vi "Compact Acquisition Software.vi"() -> ()   [LabVIEW 2022 SP3]
uses:
  Controls/All Notifer.ctl
  Controls/UI Data.ctl
  Controls/Config.ctl
  Controls/Root path.ctl
  Controls/All Loop Status.ctl
  9a3150e6-56cf-486d-8976-296f0c56f58a.vi
  f5995a21-5467-4d79-ba42-6401d0487c2b.vi
  b49e865f-9608-438f-8b3f-50d1ceeb6397.vi
  2ab09cd3-f6ad-46c6-8934-8ba6e9181128.vi
  0b75de06-b87c-40eb-ad5f-27e6ba161dd7.vi
  df10829c-ba2f-467a-a207-c0f13a0d0a80.vi
  Sub VI's/Global 1.vi
  <vilib>/Utility/TDMS File Viewer/NI_TDMS File Viewer.lvlib
panel:
  out "trans2":bool
  in  "AO Tab":enum32{"Page 1", "Page 2"}(tab)
  in  "AO_1":dbl
  in  "AO_2":dbl min=-10.0 max=10.0
  in  "AO_3":dbl
  in  "AO_4":dbl
  in  "AO_5":dbl
  in  "AO_6":dbl
  in  "AO_7":dbl caption="AO_3"
  in  "AO_8":dbl caption="AO_4"
  in  "Exit":bool
  out "transparent":bool
  in  "Tab Control":T1(tab)
  in  "tdms":bool
  in  "SEQ":bool
  in  "File transfer":T2={"File status"=FALSE, "sent file"=FALSE, "Remote Path"="/home/lvuser/natinst/bin/startup.rtexe", "Password"="", "user@host"="admin@1.1.1.4", "Local File Path"=path ""}
  in  "Enter Time(period)":dbl=15.0 format="%#_g min"
  in  "Target IP Address:":string="169.254.219.4"
  in  "RT connect":bool
  out "Device Name":string
  in  "*Select Hardware Configuration File":string(combo)
  in  "Activate Task":T3
  out "ACC,TC,SG 2":waveform(dbl)[](graph) caption="PT & RTD"
  out "ACC,TC,SG":waveform(dbl)[](graph) caption="Thermocouple Graph"
  out "HSS 10":bool
  out "HSS 9":bool
  out "HSS 8":bool
  out "HSS 7":bool
  out "HSS 6":bool
  out "HSS 5":bool
  out "HSS 4":bool
  out "HSS 3":bool
  out "HSS 2":bool
  out "HSS 1":bool
  in  "Valve_10":bool caption="EPV_10"
  in  "Valve_ 9":bool caption="EPV_9"
  in  "Valve_ 8":bool caption="EPV_8"
  in  "Valve_ 7":bool caption="EPV_7"
  in  "Valve_ 6":bool caption="EPV_6"
  in  "Valve_ 5":bool caption="EPV_5"
  in  "Valve_ 4":bool caption="EPV_4"
  in  "Valve_ 3":bool caption="EPV_3"
  in  "Valve_ 2":bool caption="EPV_2"
  in  "Valve_1":bool
  out "AI_ 10":dbl caption="AI_10" format="%#.3g bar"
  out "AI_ 9":dbl caption="AI_9" format="%#.3g bar"
  out "AI_ 8":dbl caption="AI_8" format="%#.3g bar"
  out "AI_ 7":dbl caption="AI_7" format="%#.3g bar"
  out "AI_ 6":dbl caption="AI_6" format="%#.3g bar"
  out "AI_ 5":dbl caption="AI_5" format="%#.3g bar"
  out "AI_ 4":dbl caption="HE_RTD_ATF_7" format="%#.3g Kelvin"
  out "AI_ 3":dbl caption="He_PT_ATF_1" format="%#.3g Volt"
  out "AI_ 2":dbl caption="M_RTD_1" format="%#.3g kelvin"
  out "AI_1":dbl caption="AI_3" format="%#.3g V"
  out "TC_10":dbl caption="CHN_10" format="%#.3g Deg C"
  out "TC_9":dbl caption="CHN_9" format="%#.3g Deg C"
  out "TC_8":dbl caption="CHN_8" format="%#.3g Deg C"
  out "TC_7":dbl caption="CHN_7" format="%#.3g Deg C"
  out "TC_6":dbl caption="CHN_6" format="%#.3g Deg C"
  out "TC_5":dbl caption="CHN_5" format="%#.3g Deg C"
  out "TC_4":dbl caption="CHN_4" format="%#.3g Deg C"
  out "TC_3":dbl caption="CHN_3" format="%#.3g Deg C"
  out "TC_2":dbl caption="CHN_2" format="%#.3g Deg C"
  out "TC1":dbl caption="CHN_1" format="%#.3g Deg C"
  in  "Select type":u16(ring) items=["Thermocouple", "Accelerometer", "Strain Gauge"]
  out "RT health":bool caption="RT Health"
  in  "Datalog Title:":string
  in  "Start DAQ":bool
  in  "Start Datalog":bool
  out "Data Logging?":bool
  out "SG":bool
  out "ACC":bool
  out "DI":bool
  out "TC":bool
  out "DO":bool
  out "AO":bool
  out "AI":bool
  out "Time Stamp":timestamp format="%<%x %.X>T"
  in  "Update AO":bool
  in  "Listbox":i32(listbox)
  out "vi reference":refnum<vi>
  # "Compact Acquisition Software Version 1.0"
  # "Agnikul Cosmos Private Ltd,Chennai."
  # "Analog outputs \n(1-4) channels)"
  # "Analog outputs \n(5-8)channels)"
  # "1.Select the task on the \"Activate task palette\" to perform the selected Acquisition.\n2.Select Hardware configuration File.\nTo create a new configuration,click on the \"Hardware configuration\"\nbutton in the left corner list.\n3.Start DAQ.\n4.Enter Datalog Name.\n5.Start Datalog."
  # "Every datalog will Restart at the user \ndefined time period.\n\"Default Restart time is 15 minutes.\""
  # "*Note:User Can configure 10 Analog inputs,8 Analog Outputs,10 Digital inputs,10 Digital Outputs\n10 Strain Gauge,10 Accelerometer and 10 Thermocouple."
  # "HOME"
  # "HARDWARE COFIGURATION"
  # "Digital Outputs & inputs\n (Max 10 channels)"
  # "Analog inputs\n(Max 10 channels)"
  # "TEST MODE"
  # "Help"
  # "Help and Support"
  # "If you have any doubts please contact us(Software development team)."
  # "Contact us"
  # "-Get in touch with us"
  # "Contact Info\nSoftware Development Team-LabVIEW\nEmail:\nVigneshwaranc@agnikul.in\nKannansolai@agnikul.in\nParikshitmandvikar@agnikul.in\nAjaikumar@agnikul.in"
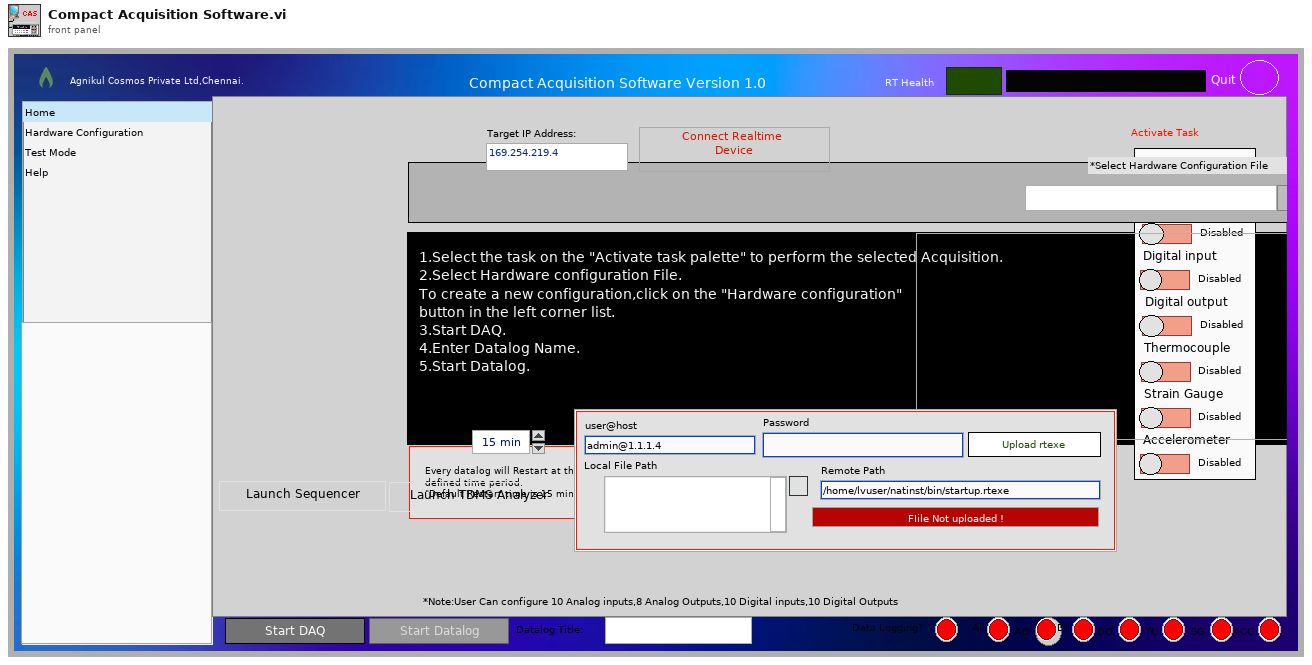
[diagram p1: front panel]
types:
  T1 = enum32{"Home Page", "Hardware Configuration", "Test Mode", "Graph View"}
  T2 = cluster{"File status":bool, "sent file":bool, "Remote Path":string, "Password":string, "user@host":string, "Local File Path":path}
  T3 = cluster{"Analog input":bool, "Analog Output":bool, "Digital input":bool, "Digital output":bool, "Thermocouple":bool, "Strain Gauge":bool, "Accelerometer":bool}
  T4 = enum32{"invalid app kind", "Development System", "Run Time System", "Student Edition", "Embedded LabVIEW", "Evaluation", "Custom"}
  T5 = typedef "All Notifer.ctl" = cluster{"UI Data":refnum<notifier>, "Start DAQ":refnum<notifier>, "Start Log":refnum<notifier>}
  T6 = typedef "Config.ctl" = cluster{"AO config":cluster{"Channel_Name":string, "Channel_Number":string, "Default_Value":dbl, "Units":string}[], "AI config":cluster{"Channel_Name":string, "Channel_Number":string, "Pre_Scale_min":dbl, "Pre_Scale_max":dbl, "Sensor_min":dbl, "Sensor_max":dbl, "Units":string}[], "DI config":cluster{"Channel_Name":string, "Channel_Number":string, "Default_Value":bool, "DI invert?":bool}[], "DO config":cluster{"Channel_Name":string, "Channel_Number":string, "Default_Value":bool, "DO invert?":bool}[], "TC config":cluster{"Channel_Name":string, "Channel_Number":string, "Pre_Scale_min":dbl, "Pre_Scale_max":dbl, "units":i32, " type":i32}[], "ACC config":cluster{"Channel_Name":string, "Channel_Number":string, "Pre_Scale_min":dbl, "Pre_Scale_max":dbl, "Terminal configuration":i32, "Sensitivity":dbl, "Sensitivity units":i32}[], "SG config":cluster{"Channel_Name":string, "Channel_Number":string, "Pre_Scale_min":dbl, "Pre_Scale_max":dbl}[], "Strain Gauge Settings":cluster{"poisson ratio":dbl, "nominal gage resistance":dbl, "gage factor":dbl}, "bridge information":cluster{"strain configuration":i32, "lead wire resistance":dbl, "initial bridge voltage":dbl, "voltage excitation source":i32, "voltage excitation value":dbl}, "Sample Rate":cluster{"AI Sample Rate":dbl, "AO Sample Rate":dbl, "DI Sample Rate":dbl, "TC Sample Rate":dbl, "DO Sample Rate":dbl, "SG Sample Rate":dbl, "ACC Sample Rate":dbl}}
  T7 = typedef "Root path.ctl" = cluster{"Data":path, "Sub VI's":path, "Source code":path}
  T8 = cluster{"notifiers ref":T5, "DAQ ref":cluster{"DI ref":refnum<vi>[], "DO ref":refnum<vi>[], "AI ref":refnum<vi>[], "AO ref":refnum<vi>[], "SG,TC,ACC":refnum<vi>[]}, "Config":T6, "NO.of.DO":u8, "NO.of.AO":u8, "user event out":refnum<user-event>, "Channel names":cluster{"AO Names":string[], "AI Names":string[], "DI Names":string[], "DO Names":string[], "TC Names":string[], "AO Default":dbl[], "DO Default":bool[], "ACC Names":string[], "SG Names":string[]}, "AO,AI,DI,DO,TC,ACC,SG":i32[], "CDAQ/CRIO(T)":bool, "DO value":bool[], "AO Value":dbl[], "Ctrl ref":cluster{"Start DAQ":refnum<vi>, "Start Log":refnum<vi>, "Tab Control":refnum<vi>}, "Root Path":T7}
  T9 = enum16{"Init", "EnQ '1'", "EnQ 'n'", "EnQ Opp", "DeQ", "Flush", "Close"}
  T10 = enum8{"Enabled", "Disabled", "Disabled and Grayed Out"}
  T11 = cluster{"no.of di":u8, "no.of ai":u8, "no.of do":u8, "no.of ao":u8, "no.of SG":u8}
  T12 = enum16{"Controls", "Transparents", "indicators", "Strings"}
  T13 = enum32{"Invalid", "Standard", "Closed", "Hidden", "Minimized", "Maximized"}
  T14 = cluster{"AO Names":string[], "AI Names":string[], "DI Names":string[], "DO Names":string[], "TC Names":string[], "AO Default":dbl[], "DO Default":bool[], "ACC Names":string[], "SG Names":string[]}
  T15 = cluster{"DI ref":refnum<vi>[], "DO ref":refnum<vi>[], "AI ref":refnum<vi>[], "AO ref":refnum<vi>[], "SG,TC,ACC":refnum<vi>[]}
  T16 = typedef "All Queue.ctl" = cluster{"AI\nAO\nDO\nTC\nACC\nStrain":refnum<queue>[], "DI":refnum<queue>}
  T17 = enum16{"Init", "Read 'All'", "Read 'n'", "Read '1'", "Write '1'", "Write 'n'", "Write 'All'"}
  T18 = cluster{"Activate Task":cluster{"Analog input":bool, "Analog Output":bool, "Digital input":bool, "Digital output":bool, "Thermocouple":bool, "Strain Gauge":bool, "Accelerometer":bool}, "Start DAQ":bool, "Start Time":timestamp, "DO Names":string[], "AO Names":string[], "AO Default":dbl[], "DO Default":bool[], "Config":cluster{"AO config":cluster{"Channel_Name":string, "Channel_Number":string, "Default_Value":dbl, "Units":string}[], "AI config":cluster{"Channel_Name":string, "Channel_Number":string, "Pre_Scale_min":dbl, "Pre_Scale_max":dbl, "Sensor_min":dbl, "Sensor_max":dbl, "Units":string}[], "DI config":cluster{"Channel_Name":string, "Channel_Number":string, "Default_Value":bool, "DI invert?":bool}[], "DO config":cluster{"Channel_Name":string, "Channel_Number":string, "Default_Value":bool, "DO invert?":bool}[], "TC config":cluster{"Channel_Name":string, "Channel_Number":string, "Pre_Scale_min":dbl, "Pre_Scale_max":dbl, "units":i32, " type":i32}[], "ACC config":cluster{"Channel_Name":string, "Channel_Number":string, "Pre_Scale_min":dbl, "Pre_Scale_max":dbl, "Terminal configuration":i32, "Sensitivity":dbl, "Sensitivity units":i32}[], "SG config":cluster{"Channel_Name":string, "Channel_Number":string, "Pre_Scale_min":dbl, "Pre_Scale_max":dbl}[], "Strain Gauge Settings":cluster{"poisson ratio":dbl, "nominal gage resistance":dbl, "gage factor":dbl}, "Bridge Settings":cluster{"voltage excitation value":dbl, "voltage excitation source":i32, "initial bridge voltage":dbl, "lead wire resistance":dbl, "strain configuration":i32}, "Sample Rate":cluster{"AI Sample Rate":dbl, "AO Sample Rate":dbl, "DI Sample Rate":dbl, "TC Sample Rate":dbl, "DO Sample Rate":dbl, "SG Sample Rate":dbl, "ACC Sample Rate":dbl}}}
  T19 = typedef "All Loop Status.ctl" = enum16{"AI", "AO", "DI", "DO", "TC", "Strain", "ACC", "RT", "Log", "Seq", "Sync"}
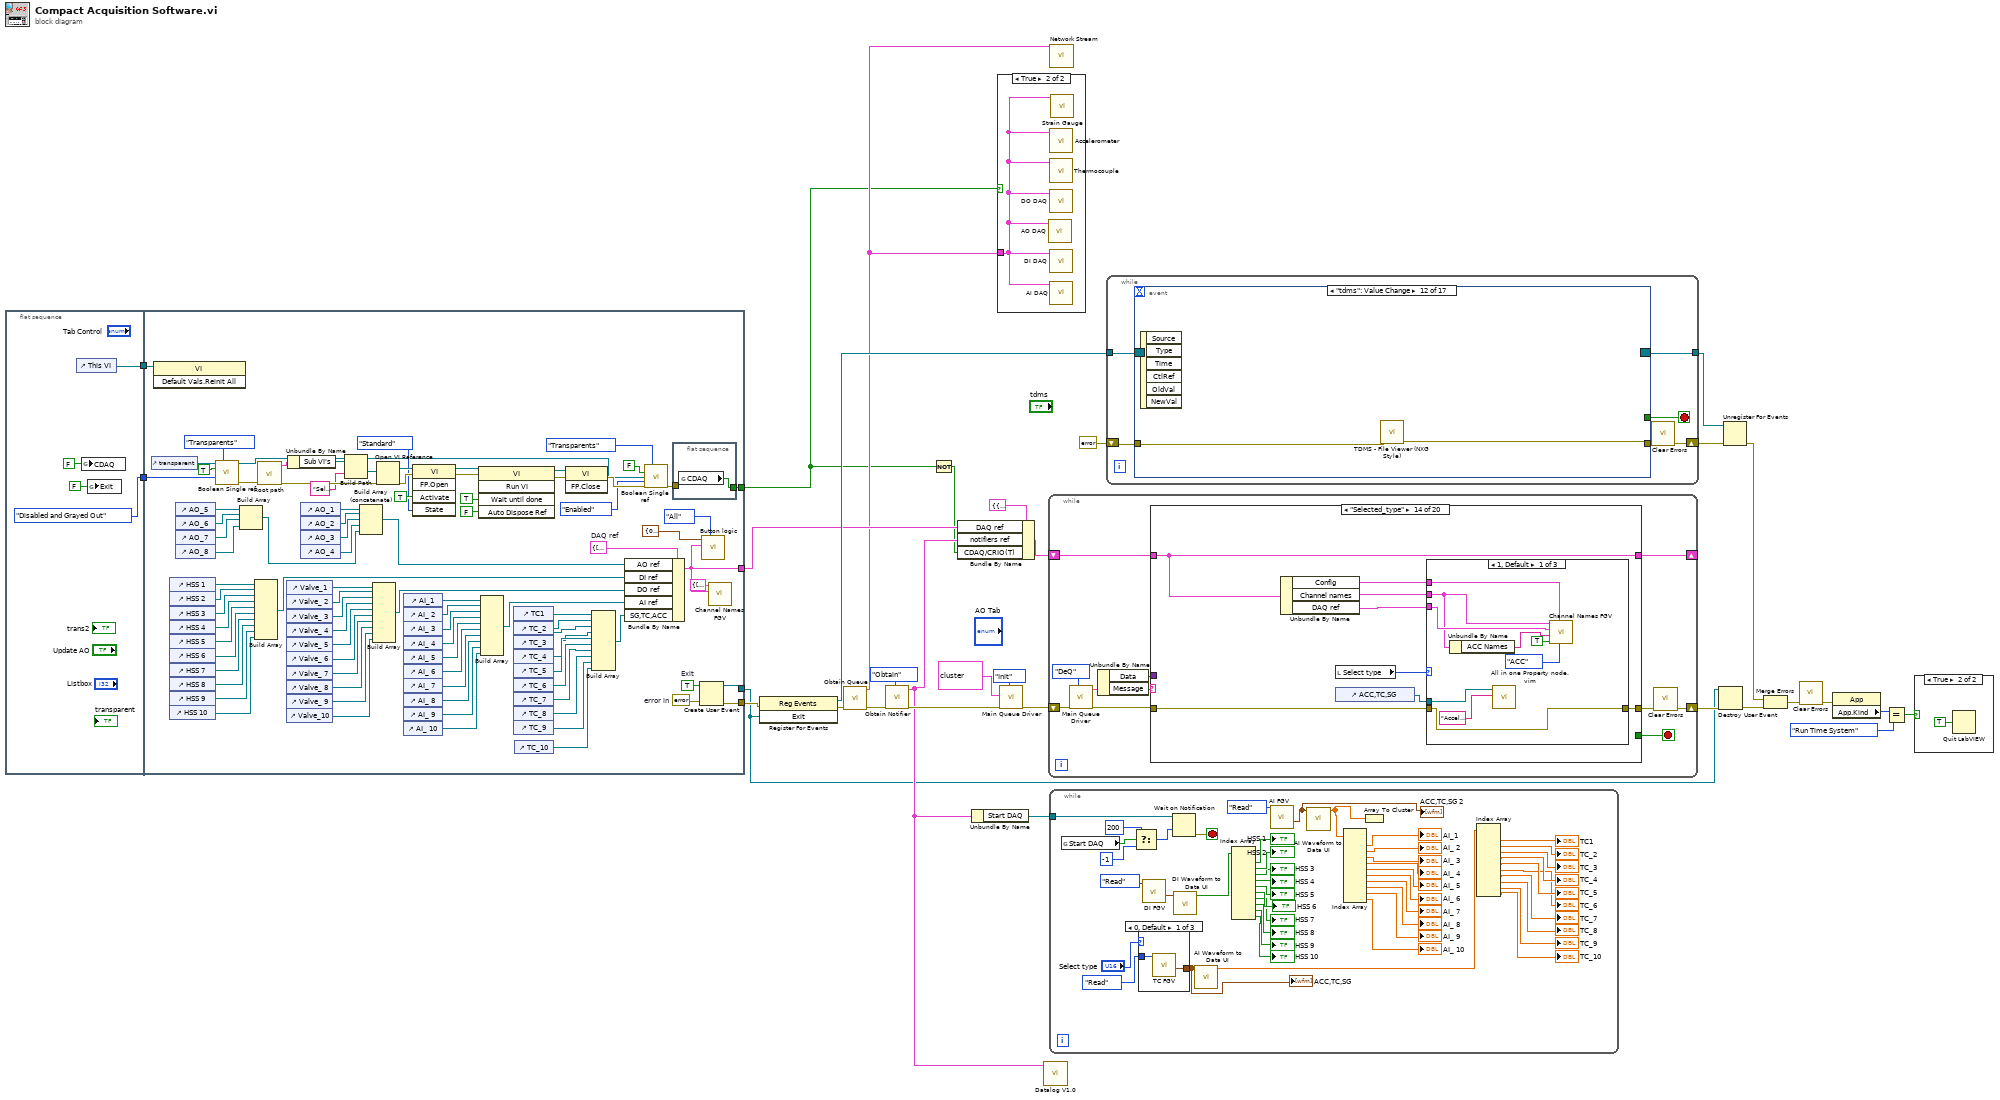
[diagram p0: block diagram]
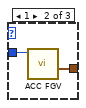
[diagram p4: hidden frame]
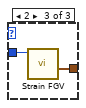
[diagram p5: hidden frame]
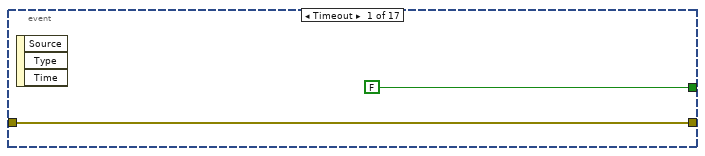
[diagram p6: hidden frame]
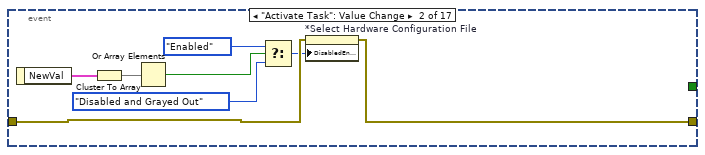
[diagram p7: hidden frame]
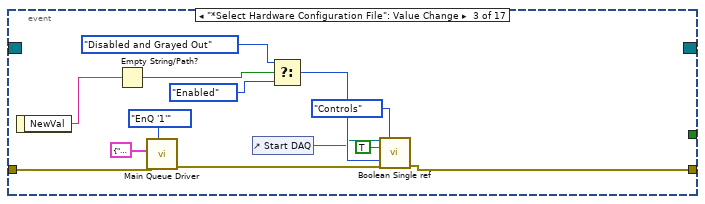
[diagram p8: hidden frame]
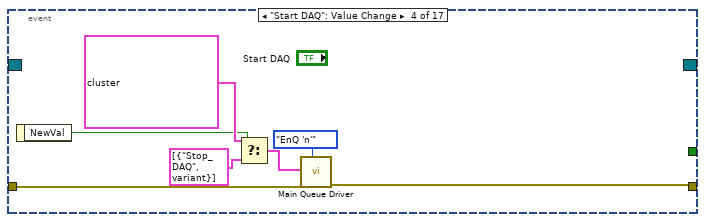
[diagram p9: hidden frame]
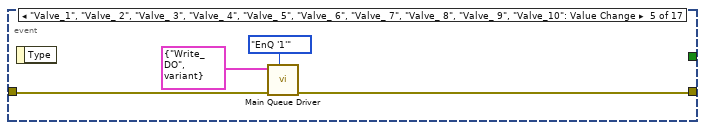
[diagram p10: hidden frame]
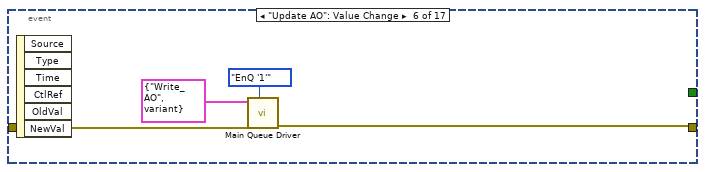
[diagram p11: hidden frame]
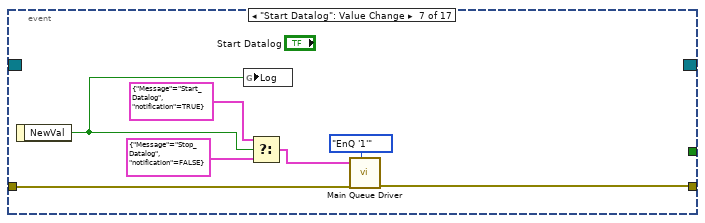
[diagram p12: hidden frame]
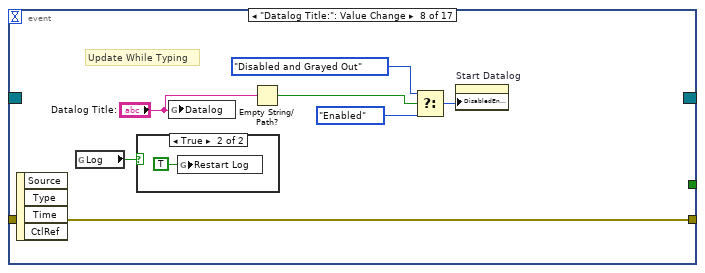
[diagram p13: hidden frame]
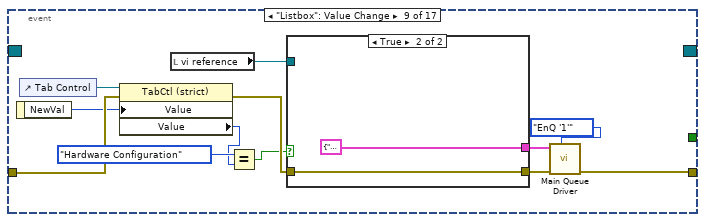
[diagram p15: hidden frame]
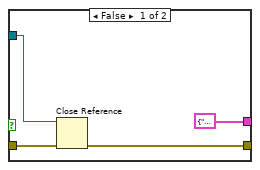
[diagram p16: hidden frame]
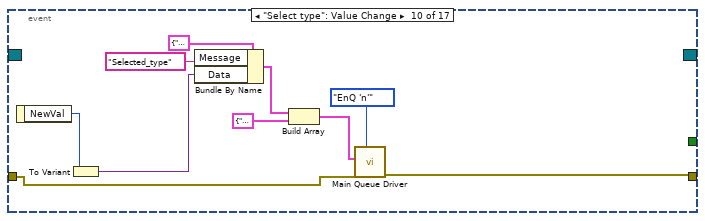
[diagram p17: hidden frame]
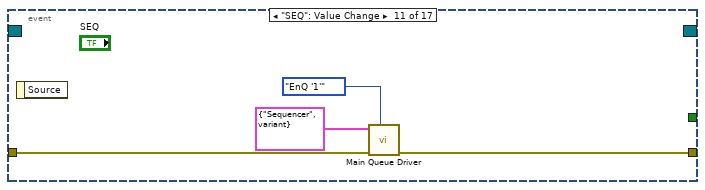
[diagram p18: hidden frame]
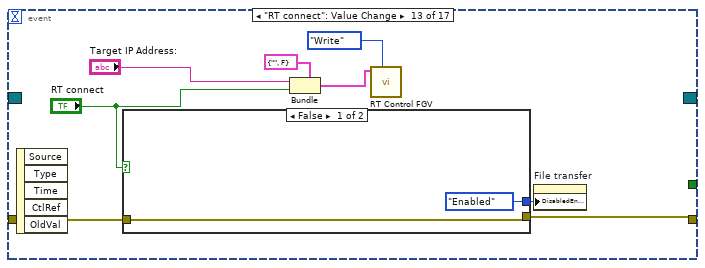
[diagram p19: hidden frame]
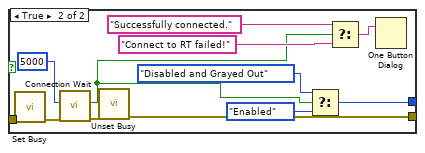
[diagram p20: hidden frame]
diagram:
  n1 = flat-sequence {
    tunnel: [w33] -> w12
    tunnel: [T10."Disabled and Grayed Out" ("Disabled")] -> w10
    tunnel: [w76] -> w18
    tunnel: [w57] -> w13
    tunnel: w12 -> [w54]
    tunnel: [w46] -> w1
    tunnel: [w45] -> w11
    tunnel: w10 -> [w43]
    frame #0 {
      n2 = control-ref of="This VI"() -> (w33:refnum<vi>)
      n3 = global write "Global 1.vi" "CDAQ"(FALSE ("CDAQ")) -> ()
      n4 = global write "Global 1.vi" "Exit"(FALSE ("Exit")) -> ()
    }
    frame #1 {
      w47 = TRUE  # Exit
      w44 = errorcluster {"status"=FALSE, "code"=0, "source"=""}  # error in
      w96 = T15 {"DI ref"=[], "DO ref"=[], "AI ref"=[], "AO ref"=[], "SG,TC,ACC"=[]}  # DAQ ref
      n5 = control-ref of="transparent"() -> (w64:refnum<vi>)
      n6 = invoke on="Invoke Node" class="VI" method="Default Vals.Reinit All"(reference=w54) -> ()  [unwired: 2 in, 3 out]
      n7 = control-ref of="HSS 1"() -> (w116:refnum<vi>)
      n8 = control-ref of="HSS 2"() -> (w115:refnum<vi>)
      n9 = control-ref of="HSS 3"() -> (w107:refnum<vi>)
      n10 = control-ref of="HSS 4"() -> (w114:refnum<vi>)
      n11 = control-ref of="HSS 5"() -> (w113:refnum<vi>)
      n12 = control-ref of="HSS 6"() -> (w112:refnum<vi>)
      n13 = control-ref of="HSS 7"() -> (w111:refnum<vi>)
      n14 = control-ref of="HSS 8"() -> (w110:refnum<vi>)
      n15 = control-ref of="HSS 9"() -> (w109:refnum<vi>)
      n16 = control-ref of="HSS 10"() -> (w108:refnum<vi>)
      n17 = control-ref of="AO_5"() -> (w40:refnum<vi>)
      n18 = control-ref of="AO_6"() -> (w39:refnum<vi>)
      n19 = control-ref of="AO_7"() -> (w38:refnum<vi>)
      n20 = control-ref of="AO_8"() -> (w37:refnum<vi>)
      n21 = call "Boolean Single ref.vi"("Enum"=T12."Transparents", "Visible"=TRUE, "trans"=w64, "Disabled"=w43) -> ("trans out"=w61:refnum<vi>, "error out"=w53:errorcluster)  [unwired: 9 in, 1 out]
      n22 = Build Array(w40, w39, w38, w37) -> (w36:refnum<vi>[])
      n23 = Build Array(w116, w115, w107, w114, w113, w112, w111, w110, w109, w108) -> (w95:refnum<vi>[])
      n24 = call "Root path.vi"("error in (no error)"=w53) -> ("error out"=w52:errorcluster, "Root Path"=w51:T7)  [unwired: 9 in]
      n25 = control-ref of="Valve_1"() -> (w126:refnum<vi>)
      n26 = control-ref of="Valve_ 2"() -> (w125:refnum<vi>)
      n27 = control-ref of="Valve_ 3"() -> (w124:refnum<vi>)
      n28 = control-ref of="Valve_ 4"() -> (w123:refnum<vi>)
      n29 = control-ref of="Valve_ 5"() -> (w122:refnum<vi>)
      n30 = control-ref of="Valve_ 6"() -> (w121:refnum<vi>)
      n31 = control-ref of="Valve_ 7"() -> (w120:refnum<vi>)
      n32 = control-ref of="Valve_ 8"() -> (w119:refnum<vi>)
      n33 = control-ref of="Valve_ 9"() -> (w118:refnum<vi>)
      n34 = control-ref of="Valve_10"() -> (w117:refnum<vi>)
      n35 = Unbundle By Name(w51) -> ("Sub VI's"=w50:path)
      n36 = control-ref of="AO_1"() -> (w92:refnum<vi>)
      n37 = control-ref of="AO_2"() -> (w91:refnum<vi>)
      n38 = control-ref of="AO_3"() -> (w90:refnum<vi>)
      n39 = control-ref of="AO_4"() -> (w89:refnum<vi>)
      n40 = Build Path(base path=w50, name or relative path="Select Device.vi") -> (appended path=w48:path)
      n41 = Build Array (concatenate)(w92, w91, w90, w89, w36) -> (w88:refnum<vi>[])
      n42 = Build Array(w126, w125, w124, w123, w122, w121, w120, w119, w118, w117) -> (w94:refnum<vi>[])
      n43 = Open VI Reference(vi path=w48, error in (no error)=w52) -> (vi reference=w69:refnum<vi>, error out=w70:errorcluster)  [unwired: 4 in]
      n44 = control-ref of="AI_1"() -> (w106:refnum<vi>)
      n45 = control-ref of="AI_ 2"() -> (w105:refnum<vi>)
      n46 = control-ref of="AI_ 3"() -> (w104:refnum<vi>)
      n47 = control-ref of="AI_ 4"() -> (w103:refnum<vi>)
      n48 = control-ref of="AI_ 5"() -> (w102:refnum<vi>)
      n49 = control-ref of="AI_ 6"() -> (w101:refnum<vi>)
      n50 = control-ref of="AI_ 7"() -> (w100:refnum<vi>)
      n51 = control-ref of="AI_ 8"() -> (w99:refnum<vi>)
      n52 = control-ref of="AI_ 9"() -> (w98:refnum<vi>)
      n53 = control-ref of="AI_ 10"() -> (w97:refnum<vi>)
      n54 = invoke on="Invoke Node" class="VI" method="FP.Open"(reference=w69, error in=w70, "Activate"=TRUE ("Activate?"), "State"=T13."Standard") -> (reference out=w71:refnum<vi>, error out=w72:errorcluster)  [unwired: 1 in, 3 out]
      n55 = invoke on="Invoke Node" class="VI" method="Run VI"(reference=w71, error in=w72, "Wait until done"=TRUE ("Wait Until Done"), "Auto Dispose Ref"=FALSE ("Auto Dispose Reference")) -> (reference out=w73:refnum<vi>, error out=w74:errorcluster)  [unwired: 1 in, 3 out]
      n56 = Build Array(w106, w105, w104, w103, w102, w101, w100, w99, w98, w97) -> (w93:refnum<vi>[])
      n57 = control-ref of="TC1"() -> (w87:refnum<vi>)
      n58 = control-ref of="TC_2"() -> (w78:refnum<vi>)
      n59 = control-ref of="TC_3"() -> (w79:refnum<vi>)
      n60 = control-ref of="TC_4"() -> (w80:refnum<vi>)
      n61 = control-ref of="TC_5"() -> (w81:refnum<vi>)
      n62 = control-ref of="TC_6"() -> (w86:refnum<vi>)
      n63 = control-ref of="TC_7"() -> (w85:refnum<vi>)
      n64 = control-ref of="TC_8"() -> (w84:refnum<vi>)
      n65 = control-ref of="TC_9"() -> (w83:refnum<vi>)
      n66 = control-ref of="TC_10"() -> (w82:refnum<vi>)
      n67 = invoke on="Invoke Node" class="VI" method="FP.Close"(reference=w73, error in=w74) -> (error out=w62:errorcluster)  [unwired: 1 in, 2 out]
      n68 = Build Array(w87, w78, w79, w80, w81, w86, w85, w84, w83, w82) -> (w77:refnum<vi>[])
      n69 = Bundle By Name(cluster=w96, "AO ref"=w88, "DI ref"=w95, "DO ref"=w94, "AI ref"=w93, "SG,TC,ACC"=w77) -> (w76:T15)
      n70 = call "Boolean Single ref.vi"("Enum"=T12."Transparents", "Visible"=FALSE, "trans"=w61, "Disabled"=T10."Enabled", "error in (no error)"=w62) -> ("error out"=w58:errorcluster)  [unwired: 8 in, 2 out]
      n71 = flat-sequence {
        tunnel: w58 -> [_]
        tunnel: [w127] -> w57
        frame #0 {
          n72 = global read "Global 1.vi" "CDAQ"() -> (w127:bool)
        }
      }
      n73 = Create User Event(user event datatype=w47, error in=w44) -> (user event=w46:refnum<user-event>, error out=w45:errorcluster)
      n74 = call "Button logic.vi"("Enum"=enum16{"DI", "AI", "DO", "All", "SG"}."All", "DAQ ref"=w76, "Cluster"=T11 {"no.of di"=0, "no.of ai"=0, "no.of do"=0, "no.of ao"=0, "no.of SG"=0}) -> ()  [unwired: 9 in]
      n75 = call "Channel Names FGV.vi"("DAQ ref"=w76, "Channel names 2"=T14 {"AO Names"=["AO_1", "AO_2", "AO_3", "AO_4"], "AI Names"=["AI_1", "AI_2", "AI_3", "AI_4", "AI_5", "AI_6", "AI_7", "AI_8", "AI_9", "AI_10"], "DI Names"=[], "DO Names"=["EPV_1", "EPV_2", "EPV_3", "EPV_4", "EPV_5", "EPV_6", "EPV_7", "EPV_8", "EPV_9", "EPV_10"], "TC Names"=["CHN_1", "CHN_2", "CHN_3", "CHN_4", "CHN_5", "CHN_6", "CHN_7", "CHN_8", "CHN_9", "CHN_10"], "AO Default"=[], "DO Default"=[], "ACC Names"=[], "SG Names"=[]}) -> ()  [unwired: 10 in]
    }
  }
  n76 = register-events(error in=w11, w1) -> (reference out=w29:refnum<event-registration>, error out=w21:errorcluster)  [unwired: 1 in]
  n77 = call "Obtain Queue.vi"("error in"=w21) -> ("error out"=w20:errorcluster, "Queue ref"=w15:T16)  [unwired: 9 in]
  n78 = call "Obtain Notifier.vi"("Case"=enum16{"Obtain", "Read"}."Obtain", "error in (no error)"=w20) -> ("error out"=w23:errorcluster, "notifiers out"=w16:T5)  [unwired: 8 in]
  n79 = Not(x=w13) -> (.not. x?=w14:bool)
  n80 = Bundle By Name(cluster=T8 {"notifiers ref"={"UI Data"=refnum, "Start DAQ"=refnum, "Start Log"=refnum}, "DAQ ref"={"DI ref"=[], "DO ref"=[], "AI ref"=[], "AO ref"=[], "SG,TC,ACC"=[]}, "Config"={"AO config"=[], "AI config"=[], "DI config"=[], "DO config"=[], "TC config"=[{"Channel_Name"="", "Channel_Number"="", "Pre_Scale_min"=0.0, "Pre_Scale_max"=0.0, "units"=4, " type"=7}], "ACC config"=[], "SG config"=[], "Strain Gauge Settings"={"poisson ratio"=0.3, "nominal gage resistance"=120.0, "gage factor"=2.08}, "bridge information"={"strain configuration"=10271, "lead wire resistance"=1.7, "initial bridge voltage"=0.0, "voltage excitation source"=10200, "voltage excitation value"=3.3}, "Sample Rate"={"AI Sample Rate"=0.0, "AO Sample Rate"=0.0, "DI Sample Rate"=0.0, "TC Sample Rate"=0.0, "DO Sample Rate"=0.0, "SG Sample Rate"=0.0, "ACC Sample Rate"=0.0}}, "NO.of.DO"=0, "NO.of.AO"=0, "user event out"=refnum, "Channel names"={"AO Names"=[], "AI Names"=[], "DI Names"=[], "DO Names"=[], "TC Names"=[], "AO Default"=[], "DO Default"=[], "ACC Names"=[], "SG Names"=[]}, "AO,AI,DI,DO,TC,ACC,SG"=[], "CDAQ/CRIO(T)"=TRUE, "DO value"=[], "AO Value"=[], "Ctrl ref"={"Start DAQ"=refnum, "Start Log"=refnum, "Tab Control"=refnum}, "Root Path"={"Data"=path "", "Sub VI's"=path "", "Source code"=path ""}}, "DAQ ref"=w18, "notifiers ref"=w16, "CDAQ/CRIO(T)"=w14) -> (w24:T8)
  n81 = Unbundle By Name(w16) -> ("Start DAQ"=w22:refnum<notifier>)
  n82 = case shown="True" w13 {
    tunnel: w15 -> [_ w128]
    frame False {
    }
    frame True {
      n83 = call "AO DAQ.vi"("Queue ref"=w128) -> ()  [unwired: 11 in]
      n84 = call "Accelerometer.vi"("Queue ref"=w128) -> ()  [unwired: 11 in]
      n85 = call "Thermocouple.vi"("Queue ref"=w128) -> ()  [unwired: 11 in]
      n86 = call "DO DAQ.vi"("Queue ref"=w128) -> ()  [unwired: 11 in]
      n87 = call "DI DAQ.vi"("Queue ref"=w128) -> ()  [unwired: 11 in]
      n88 = call "AI DAQ.vi"("Queue ref"=w128) -> ()  [unwired: 11 in]
      n89 = call "Strain Gauge.vi"("Queue ref"=w128) -> ()  [unwired: 11 in]
    }
  }
  n90 = call "Main Queue Driver.vi"("Option"=T9."Init", "error in (no error)"=w23, "Messages"=cluster{"Message":string, "Data":variant}[] [{"Message"="Initialize", "Data"=variant}, {"Message"="Login", "Data"=variant}, {"Message"="Refresh_files", "Data"=variant}]) -> ("error out"=w31:errorcluster)  [unwired: 7 in, 1 out]
  n91 = call "Datalog V1.0.vi"("notifiers in"=w16) -> ()  [unwired: 11 in]
  n92 = while {
    shift-right: [w139] -> w27
    shift-left: w31 -> [w131]
    shift-right: [w132] -> _
    shift-left: w24 -> [w133]
    stop <- w137 stop-if-true
    n93 = call "Main Queue Driver.vi"("Option"=T9."DeQ", "error in (no error)"=w131) -> ("error out"=w130:errorcluster, "Message Out"=w135:cluster{"Message":string, "Data":variant})  [unwired: 8 in]
    n94 = Unbundle By Name(w135) -> ("Data"=w129:variant, "Message"=w134:string)
    n95 = case shown="\"Selected_type\"" w134 {
      tunnel: w130 -> [w144 w166 w186 w207 w213 w233 w257 w271 w311 w324 w337 w369 w394 w402 w435 w441 w453 w458 w459 w478]
      tunnel: [w143 w163 w186 w207 w212 w225 w246 w268 w312 w325 w338 w367 w394 w401 w432 w440 w456 w458 w460 w480] -> w138
      tunnel: [_ FALSE _ _ _ _ _ _ _ _ _ _ _ _ _ _ _ _ _ TRUE] -> w137
      tunnel: w133 -> [w142 w176 w200 w206 w211 w218 w250 w265 w318 w330 w341 w370 w391 w399 w436 w438 w455 w457 w470 w484]
      tunnel: [w142 w180 w199 w206 w211 w227 w253 w266 w318 w330 w339 w371 w389 w399 w436 w438 w455 w457 w470 w484] -> w132
      tunnel: w129 -> [_ _ _ _ _ _ _ _ _ _ _ _ _ _ _ _ w451 _ _ _]
      frame "pollevent", Default {
        w156 = T19[] [enum."AI", enum."AO", enum."DI", enum."DO", enum."TC", enum."ACC", enum."Strain", enum."Log", enum."RT"] items=["AI", "AO", "DI", "DO", "TC", "Strain", "ACC", "RT", "Log", "Seq", "Sync"] ("Loops")
        n96 = Unbundle By Name(w142) -> ("DAQ ref.DO ref"=w141:refnum<vi>[], "DAQ ref.AO ref"=w140:refnum<vi>[])
        n97 = call "ALS Feedback DO ref.vi"("DAQ ref.AO ref"=w140, "DAQ ref.DO ref"=w141) -> ()  [unwired: 10 in]
        n98 = call "ALL Loop Status.vi"("Option"=T17."Read 'n'", "error in (no error)"=w144, "Loops"=w156) -> ("error out"=w143:errorcluster, "Status List Out"=w155:bool[])  [unwired: 6 in, 1 out]
        n99 = Index Array(array=w155) -> (element #1=→"AI":bool, element #2=→"AO":bool, element #3=→"DI":bool, element #4=→"DO":bool, element #5=→"TC":bool, element #6=→"ACC":bool, element #7=→"SG":bool, element #8=→"Data Logging?":bool, element #9=→"RT health":bool)  [unwired: 9 in]
        n100 = Get Date/Time In Seconds() -> (seconds since 1Jan1904=→"Time Stamp":timestamp)
      }
      frame "Initialize" {
        n101 = Unbundle By Name(w176) -> ("CDAQ/CRIO(T)"=w159:bool)
        n102 = property on="Listbox" class="LstBox (strict)"(error in=w166, "Item Names"=string[] ["Home", "Hardware Configuration", "Test Mode", "Help"]) -> (error out=w165:errorcluster)  [unwired: 1 in, 1 out]
        n103 = Select(t="Ready to Start Acquisition in Realtime (cRIO)" ("Device Name"), s=w159, f="Ready to Start Acquisition in cDAQ" ("Device Name")) -> (s? t:f=→"Device Name":string)
        n104 = control-ref of="RT health"() -> (w174:refnum<vi>)
        n105 = control-ref of="RT connect"() -> (w173:refnum<vi>)
        n106 = control-ref of="Target IP Address:"() -> (w160:refnum<vi>)
        n107 = global write "Global 1.vi" "ALS"(FALSE ("CDAQ")) -> ()
        n108 = Build Array(w174, w173, w160) -> (w172:refnum<vi>[])
        n109 = call "ALL Loop Status.vi"("Option"=T17."Init", "error in (no error)"=w165) -> ("error out"=w178:errorcluster)  [unwired: 7 in, 2 out]
        n110 = call "All in one Property node.vim"("Visible(T)/Value(F)"=TRUE ("Value(F)"), "Boolean"=w159, "ref in"=w172) -> ()  [unwired: 7 in, 2 out]
        n111 = property on="File transfer" class="Clust"("Visible"=w159) -> ()  [unwired: 2 in, 2 out]
        n112 = call "Root path.vi"("error in (no error)"=w178) -> ("error out"=w177:errorcluster, "Root Path"=w175:T7)  [unwired: 9 in]
        n113 = control-ref of="*Select Hardware Configuration File"() -> (w168:refnum<vi>)
        n114 = control-ref of="Tab Control"() -> (w179:refnum<vi>)
        n115 = control-ref of="Start DAQ"() -> (w171:refnum<vi>)
        n116 = control-ref of="Start Datalog"() -> (w170:refnum<vi>)
        n117 = property on="trans2" class="Bool (strict)"("Visible"=TRUE) -> ()  [unwired: 2 in, 2 out]
        n118 = Bundle By Name(cluster=w176, "Root Path"=w175, "Ctrl ref.Start DAQ"=w171, "Ctrl ref.Start Log"=w170, "Ctrl ref.Tab Control"=w179) -> (w180:T8)
        n119 = Build Array(w171, w170, w168) -> (w169:refnum<vi>[])
        n120 = call "All in one Property node.vim"("error in (no error)"=w177, "Boolean"=T10."Disabled and Grayed Out", "ref in"=w169) -> ("error out"=w163:errorcluster)  [unwired: 7 in, 1 out]
      }
      frame "Button Logic" {
        n121 = local read "Select type"() -> (w190:u16)
        n122 = Unbundle By Name(w200) -> ("DAQ ref"=w201:T15, "AO,AI,DI,DO,TC,ACC,SG"=w188:i32[])
        n123 = case shown="0" w190 {
          tunnel: [4 ("index") 5 ("index") 6 ("index")] -> w189
          frame 0 {
          }
          frame 1 {
          }
          frame 2, Default {
          }
        }
        n124 = To Unsigned Byte Integer(number=w188) -> (unsigned 8bit integer=w187:u8[])
        n125 = Index Array(array=w187, index #1=1 ("index"), index #5=w189) -> (element #1=w195:u8, element #2=w198:u8, element #3=w197:u8, element #4=w196:u8, element #5=w191:u8)  [unwired: 3 in]
        n126 = Bundle By Name(cluster=T11 {"no.of di"=0, "no.of ai"=0, "no.of do"=0, "no.of ao"=0, "no.of SG"=0} ("Cluster"), "no.of ao"=w195, "no.of ai"=w198, "no.of di"=w197, "no.of do"=w196, "no.of SG"=w191) -> (w202:T11)
        n127 = call "Button logic.vi"("Enum"=enum16{"DI", "AI", "DO", "All", "SG"}."All", "DAQ ref"=w201, "Cluster"=w202) -> ()  [unwired: 9 in]
        n128 = Bundle By Name(cluster=w200, "NO.of.DO"=w196, "NO.of.AO"=w195) -> (w199:T8)
      }
      frame "Login" {
      }
      frame "Refresh_files" {
        n129 = Unbundle By Name(w211) -> ("Root Path.Data"=w210:path)
        n130 = Build Path(base path=w210, name or relative path=path "HW config") -> (appended path=w208:path)
        n131 = List Folder(path=w208, error in=w213) -> (filenames=w215:string[], error out=w214:errorcluster)  [unwired: 2 in, 2 out]
        n132 = property on="*Select Hardware Configuration File" class="CmbBox"(error in=w214, "Strings[]"=w215) -> (error out=w212:errorcluster)  [unwired: 1 in, 1 out]
      }
      frame "Hardware_config" {
        n133 = Unbundle By Name(w218) -> ("Root Path.Sub VI's"=w217:path)
        n134 = Build Path(base path=w217, name or relative path=path "Hardware Config.vi") -> (appended path=w216:path)
        n135 = Open VI Reference(vi path=w216, error in (no error)=w233) -> (vi reference=w229:refnum<vi>, error out=w231:errorcluster)  [unwired: 4 in]
        "vi reference" <- w229
        n136 = flat-sequence {
          tunnel: [w239] -> w226
          tunnel: [w237] -> w220
          tunnel: w221 -> [w234]
          frame #0 {
            n137 = global read "Global 1.vi" "Hw file"() -> (w236:string)
            n138 = Empty String/Path?(string/path=w236) -> (empty?=w235:bool)
            n139 = case shown="False" w235 {
              tunnel: w236 -> [w243 _]
              tunnel: [w242 w244] -> w238
              tunnel: w234 -> [w241 w244]
              frame False {
                n140 = property on="*Select Hardware Configuration File" class="CmbBox"(error in=w241, "Val(Sgnl)"=w243) -> (error out=w242:errorcluster)  [unwired: 1 in, 1 out]
              }
              frame True {
              }
            }
            n141 = call "Config FGV.vi"("Enum"=enum16{"Read", "Write"}."Read", "error in (no error)"=w238) -> ("error out"=w237:errorcluster, "Data"=w239:T6)  [unwired: 8 in]
          }
        }
        n142 = invoke on="Sub Panel" class="SubPnl" method="Insert VI"(error in=w231, "VI Ref"=w229) -> (error out=w228:errorcluster)  [unwired: 2 in, 3 out]
        n143 = invoke on="Invoke Node" class="VI" method="Run VI"(reference=w229, error in=w228, "Wait until done"=FALSE ("Wait Until Done"), "Auto Dispose Ref"=FALSE ("Auto Dispose Reference")) -> (error out=w221:errorcluster)  [unwired: 1 in, 4 out]
        n144 = call "Main Queue Driver.vi"("Option"=T9."EnQ '1'", "Message"=cluster{"Message":string, "Data":variant} {"Message"="Refresh_files", "Data"=variant}) -> ("error out"=w224:errorcluster)  [unwired: 8 in, 1 out]
        n145 = Bundle By Name(cluster=w218, "Config"=w226) -> (w227:T8)
        n146 = Merge Errors(w220, w224, w221) -> (w225:errorcluster)
      }
      frame "Load_Config" {
        n147 = Unbundle By Name(w250) -> ("Root Path.Data"=w249:path)
        n148 = Build Path(base path=w249, name or relative path=path "HW config" ("Select Hardware Configuration File to Start DAQ")) -> (appended path=w247:path)
        n149 = Build Path(base path=w247, name or relative path="*Select Hardware Configuration File") -> (appended path=w251:path)
        n150 = call "Load Config.vi"("error in"=w257, "file path (use dialog)"=w251) -> ("error out"=w255:errorcluster, "data"=w254:T6)  [unwired: 8 in]
        n151 = call "Config FGV.vi"("Enum"=enum16{"Read", "Write"}."Write", "error in (no error)"=w255, "Data 2"=w254) -> ("error out"=w246:errorcluster, "Data"=w245:T6)  [unwired: 7 in]
        n152 = Bundle By Name(cluster=w250, "Config"=w245) -> (w253:T8)
      }
      frame "Start_DAQ" {
        n153 = Unbundle By Name(w265) -> ("CDAQ/CRIO(T)"=w264:bool, "Config"=w263:T6, "AO Value"=w262:dbl[], "DO value"=w261:bool[], "Ctrl ref.Tab Control"=w259:refnum<vi>)
        n154 = global write "Global 1.vi" "Start DAQ"(TRUE ("Start DAQ")) -> ()
        n155 = local write "Listbox"(2 ("Listbox")) -> ()
        n156 = property on="trans2" class="Bool (strict)"("Visible"=FALSE) -> ()  [unwired: 2 in, 2 out]
        n157 = call "All Channel Names.vi"("Enum"=enum16{"Read", "Write"}."Read") -> ("Channel names"=w270:T14)  [unwired: 13 in, 1 out]
        n158 = case shown="True" w264 {
          tunnel: "Activate Task" -> [w287 w305]
          tunnel: w265 -> [w275 w295]
          tunnel: w271 -> [w283 w307]
          tunnel: w270 -> [w282 w306]
          tunnel: [w278 w294] -> w268
          tunnel: [w275 w295] -> w266
          tunnel: w263 -> [_ w298]
          tunnel: w262 -> [_ w297]
          tunnel: w261 -> [_ w296]
          tunnel: w259 -> [w273 w290]
          frame False {
            w285 = enum16{"Read", "Write", "Start time", "init"}."Start time" ("Enum")
            n159 = Unbundle By Name(w282) -> ("DO Names"=w280:string[], "AO Names"=w281:string[])
            n160 = call "Activated TAsk.vi"("Enum"=enum16{"Read", "Write"}."Write", "error in (no error)"=w283, "Activate Task"=w287) -> ("error out"=w279:errorcluster, "Start Time"=w284:timestamp)  [unwired: 6 in, 1 out]
            n161 = Unbundle By Name(w275) -> ("notifiers ref.Start DAQ"=w277:refnum<notifier>)
            n162 = call "AO FGV.vi"("Enum"=w285, "Start Time"=w284, "AO Channel Names"=w281) -> ()  [unwired: 7 in, 2 out]
            n163 = property on="Property Node" class="TabCtl (strict)"(reference=w273, "Value"=T1."Test Mode") -> ()  [unwired: 1 in, 2 out]
            n164 = call "DO FGV.vi"("Enum"=w285, "Start Time"=w284, "DO Channel Names"=w280) -> ()  [unwired: 6 in, 3 out]
            n165 = Send Notification(notification=TRUE, notifier=w277, error in (no error)=w279) -> (error out=w278:errorcluster)  [unwired: 1 out]
          }
          frame True {
            # "RT DAQ"
            n166 = Unbundle By Name(w306) -> ("DO Names"=w304:string[], "AO Names"=w303:string[])
            n167 = Get Date/Time In Seconds() -> (seconds since 1Jan1904=w302:timestamp)
            n168 = Add(x=w302, y=5.0) -> (x+y=w300:timestamp)
            n169 = Bundle By Name(cluster=T18 {"Activate Task"={"Analog input"=TRUE, "Analog Output"=TRUE, "Digital input"=TRUE, "Digital output"=TRUE, "Thermocouple"=FALSE, "Strain Gauge"=TRUE, "Accelerometer"=TRUE}, "Start DAQ"=TRUE, "Start Time"=timestamp(0 s since 1904-01-01), "DO Names"=[], "AO Names"=[], "AO Default"=[], "DO Default"=[], "Config"={"AO config"=[], "AI config"=[], "DI config"=[], "DO config"=[], "TC config"=[{"Channel_Name"="", "Channel_Number"="", "Pre_Scale_min"=0.0, "Pre_Scale_max"=0.0, "units"=4, " type"=7}], "ACC config"=[], "SG config"=[], "Strain Gauge Settings"={"poisson ratio"=0.3, "nominal gage resistance"=120.0, "gage factor"=2.08}, "Bridge Settings"={"voltage excitation value"=3.3, "voltage excitation source"=10200, "initial bridge voltage"=0.0, "lead wire resistance"=1.7, "strain configuration"=10271}, "Sample Rate"={"AI Sample Rate"=0.0, "AO Sample Rate"=0.0, "DI Sample Rate"=0.0, "TC Sample Rate"=0.0, "DO Sample Rate"=0.0, "SG Sample Rate"=0.0, "ACC Sample Rate"=0.0}}}, "DO Names"=w304, "AO Names"=w303, "Activate Task"=w305, "Start Time"=w300, "Start DAQ"=TRUE, "Config"=w298, "AO Default"=w297, "DO Default"=w296) -> (w310:T18)
            n170 = property on="Property Node" class="TabCtl (strict)"(reference=w290, "Value"=T1."Test Mode") -> ()  [unwired: 1 in, 2 out]
            n171 = Unbundle By Name(w295) -> ("notifiers ref.Start DAQ"=w291:refnum<notifier>)
            n172 = To Variant(anything=w310) -> (Variant=w309:variant)
            n173 = call "Networkstream UI Command.vi"("error in"=w307, "Data"=w309, "Message"="Start DAQ") -> ("error out"=w293:errorcluster)  [unwired: 8 in]
            n174 = Send Notification(notification=TRUE ("ignore previous (F)"), notifier=w291, error in (no error)=w293) -> (error out=w294:errorcluster)  [unwired: 1 out]
          }
        }
      }
      frame "Update_DO" {
        n175 = Unbundle By Name(w318) -> ("DAQ ref.DO ref"=w317:refnum<vi>[])
        n176 = call "All Channel Names.vi"("Enum"=enum16{"Read", "Write"}."Read") -> ("Channel names"=w315:T14)  [unwired: 13 in, 1 out]
        n177 = Unbundle By Name(w315) -> ("DO Default"=w314:bool[])
        n178 = for {
          tunnel: w317 -> [w321] mode=indexing
          tunnel: [w322] -> w313 mode=indexing
          tunnel: w314 -> [w320] mode=indexing
          tunnel: w311 -> [w319]
          n179 = call "All in one Property node.vim"("error in (no error)"=w319, "Boolean"=w320, "ref in"=w321) -> ("error out"=w322:errorcluster)  [unwired: 7 in, 1 out]
        }
        n180 = Merge Errors(w313, w311) -> (w312:errorcluster)
      }
      frame "Update_AO" {
        n181 = Unbundle By Name(w330) -> ("DAQ ref.AO ref"=w329:refnum<vi>[])
        n182 = call "All Channel Names.vi"("Enum"=enum16{"Read", "Write"}."Read") -> ("Channel names"=w327:T14)  [unwired: 13 in, 1 out]
        n183 = Unbundle By Name(w327) -> ("AO Default"=w326:dbl[])
        n184 = for {
          tunnel: w329 -> [w334] mode=indexing
          tunnel: w326 -> [w331] mode=indexing
          tunnel: w324 -> [w332]
          tunnel: [w333] -> w323 mode=indexing
          n185 = property class="DigNum (strict)"(reference=w334, error in=w332, "Value"=w331) -> (error out=w333:errorcluster)  [unwired: 1 out]
        }
        n186 = Merge Errors(w323, w324) -> (w325:errorcluster)
      }
      frame "Write_DO" {
        n187 = Unbundle By Name(w341) -> ("NO.of.DO"=w343:u8, "CDAQ/CRIO(T)"=w336:bool)
        n188 = To Long Integer(number=w343) -> (32bit integer=w342:i32)
        n189 = Build Array("Valve_1", "Valve_ 2", "Valve_ 3", "Valve_ 4", "Valve_ 5", "Valve_ 6", "Valve_ 7", "Valve_ 8", "Valve_ 9", "Valve_10") -> (w345:bool[])
        n190 = Array Subset(array=w345, length=w342) -> (w340:bool[])  [unwired: 1 in]
        n191 = call "DO FGV.vi"("Enum"=enum16{"Read", "Write", "Start time", "init"}."Write", "DO in"=w340) -> ("DO out"=w335:bool[])  [unwired: 7 in, 2 out]
        n192 = case shown="True" w336 {
          tunnel: w337 -> [w356 w360]
          tunnel: [w356 w361] -> w338
          tunnel: w335 -> [_ w357]
          frame False {
          }
          frame True {
            n193 = To Variant(anything=w357) -> (Variant=w358:variant)
            n194 = call "Networkstream UI Command.vi"("error in"=w360, "Data"=w358, "Message"="Write_DO") -> ("error out"=w361:errorcluster)  [unwired: 8 in]
          }
        }
        n195 = Bundle By Name(cluster=w341, "DO value"=w335) -> (w339:T8)
      }
      frame "Write_AO" {
        n196 = Unbundle By Name(w370) -> ("NO.of.AO"=w376:u8, "CDAQ/CRIO(T)"=w366:bool)
        n197 = To Long Integer(number=w376) -> (32bit integer=w374:i32)
        n198 = Build Array("AO_1", "AO_2", "AO_3", "AO_4", "AO_5", "AO_6", "AO_7", "AO_8") -> (w375:dbl[])
        n199 = Array Subset(array=w375, length=w374) -> (w373:dbl[])  [unwired: 1 in]
        n200 = call "AO FGV.vi"("Enum"=enum16{"Read", "Write", "Start time", "init"}."Write", "AO in"=w373) -> ("AO out"=w368:dbl[])  [unwired: 8 in, 1 out]
        n201 = Bundle By Name(cluster=w370, "AO Value"=w368) -> (w371:T8)
        n202 = case shown="True" w366 {
          tunnel: w369 -> [w381 w385]
          tunnel: [w381 w386] -> w367
          tunnel: w368 -> [_ w382]
          frame False {
          }
          frame True {
            n203 = To Variant(anything=w382) -> (Variant=w383:variant)
            n204 = call "Networkstream UI Command.vi"("error in"=w385, "Data"=w383, "Message"="Write_AO") -> ("error out"=w386:errorcluster)  [unwired: 8 in]
          }
        }
      }
      frame "Rename_Label" {
        n205 = Unbundle By Name(w391) -> ("Config"=w387:T6, "DAQ ref"=w392:T15)
        n206 = call "All Channel Names.vi"("Data"=w387, "Enum"=enum16{"Read", "Write"}."Write") -> ("Channel names"=w390:T14, "AO,AI,DI,DO,TC,ACC,SG"=w388:i32[])  [unwired: 12 in]
        n207 = call "Channel Names FGV.vi"("Config"=w387, "DAQ ref"=w392, "Channel names 2"=w390) -> ()  [unwired: 9 in]
        n208 = Bundle By Name(cluster=w391, "Channel names"=w390, "AO,AI,DI,DO,TC,ACC,SG"=w388) -> (w389:T8)
      }
      frame "Selected_type" {
        n209 = Unbundle By Name(w399) -> ("Config"=w395:T6, "Channel names"=w396:T14, "DAQ ref"=w398:T15)
        n210 = local read "Select type"() -> (w397:u16)
        n211 = control-ref of="ACC,TC,SG"() -> (w400:refnum<vi>)
        n212 = case shown="1, Default" w397 {
          tunnel: w402 -> [w411 w420 w429]
          tunnel: [w411 w420 w429] -> w401
          tunnel: w400 -> [w404 w413 w422]
          tunnel: w396 -> [w407 w417 w425]
          tunnel: w398 -> [w408 w418 w426]
          tunnel: w395 -> [w406 w414 w423]
          frame 1, Default {
            n213 = Unbundle By Name(w407) -> ("ACC Names"=w409:string[])
            n214 = call "All in one Property node.vim"("Boolean"="Accelerometer Graph" ("Caption.Text"), "ref in"=w404) -> ()  [unwired: 8 in, 2 out]
            n215 = call "Channel Names FGV.vi"("type"=enum16{"TC", "ACC", "SG"}."ACC", "Config"=w406, "t"=TRUE, "names"=w409, "DAQ ref"=w408, "Channel names 2"=w407) -> ()  [unwired: 6 in]
          }
          frame 0 {
            n216 = Unbundle By Name(w417) -> ("TC Names"=w416:string[])
            n217 = call "All in one Property node.vim"("Boolean"="Thermocouple Graph" ("Caption.Text"), "ref in"=w413) -> ()  [unwired: 8 in, 2 out]
            n218 = call "Channel Names FGV.vi"("type"=enum16{"TC", "ACC", "SG"}."TC", "Config"=w414, "t"=TRUE, "names"=w416, "DAQ ref"=w418, "Channel names 2"=w417) -> ()  [unwired: 6 in]
          }
          frame 2 {
            n219 = Unbundle By Name(w425) -> ("SG Names"=w427:string[])
            n220 = call "All in one Property node.vim"("Boolean"="Strain Gauge Graph" ("Caption.Text"), "ref in"=w422) -> ()  [unwired: 8 in, 2 out]
            n221 = call "Channel Names FGV.vi"("type"=enum16{"TC", "ACC", "SG"}."SG", "Config"=w423, "t"=TRUE, "names"=w427, "DAQ ref"=w426, "Channel names 2"=w425) -> ()  [unwired: 6 in]
          }
        }
      }
      frame "RTD_graph" {
        n222 = Unbundle By Name(w436) -> ("Config"=w434:T6)
        n223 = call "RTD and PT index split.vi"("error in (no error)"=w435, "config"=w434) -> ("error out"=w433:errorcluster, "RTD"=w431:i32[])  [unwired: 8 in]
        n224 = control-ref of="ACC,TC,SG 2"() -> (w430:refnum<vi>)
        n225 = call "Duplicate y Scale.vi"("error in (no error)"=w433, "Plot.Y Scale Index"=w431, "ACC,TC,SG 2"=w430) -> ("error out"=w432:errorcluster)  [unwired: 8 in]
      }
      frame "Stop_DAQ" {
        n226 = Unbundle By Name(w438) -> ("CDAQ/CRIO(T)"=w437:bool)
        n227 = global write "Global 1.vi" "Start DAQ"(FALSE ("Start DAQ")) -> ()
        n228 = case shown="False" w437 {
          tunnel: w441 -> [w443 w446]
          tunnel: [w443 w445] -> w440
          frame False {
          }
          frame True {
            n229 = To Variant(anything=TRUE ("Visible")) -> (Variant=w448:variant)
            n230 = call "Networkstream UI Command.vi"("error in"=w446, "Data"=w448, "Message"="Stop DAQ") -> ("error out"=w445:errorcluster)  [unwired: 8 in]
          }
        }
        n231 = property on="trans2" class="Bool (strict)"("Visible"=TRUE) -> ()  [unwired: 2 in, 2 out]
      }
      frame "Start_Datalog" {
        n232 = Unbundle By Name(w455) -> ("notifiers ref.Start Log"=w454:refnum<notifier>)
        n233 = Variant To Data(error in=w453, type=FALSE ("notification"), Variant=w451) -> (data=w449:bool, error out=w452:errorcluster)
        n234 = Send Notification(notification=w449, notifier=w454, error in (no error)=w452) -> (error out=w456:errorcluster)  [unwired: 1 out]
      }
      frame "Stop_Datalog" {
      }
      frame "Sequencer" {
        # "M:\\Sequencer Test Bench\\Source code\\Sequencer"
        n235 = Unbundle By Name(w470) -> ("Root Path.Source code"=w469:path)
        n236 = Build Path(base path=w469, name or relative path=path "Sequencer/Sequencer Main.vi") -> (appended path=w471:path)
        n237 = Open VI Reference(vi path=w471, error in (no error)=w459) -> (vi reference=w468:refnum<vi>, error out=w463:errorcluster)  [unwired: 4 in]
        n238 = invoke on="Invoke Node" class="VI" method="FP.Open"(reference=w468, error in=w463, "Activate"=TRUE ("Activate?"), "State"=T13."Standard") -> (reference out=w462:refnum<vi>, error out=w461:errorcluster)  [unwired: 1 in, 3 out]
        n239 = invoke on="Invoke Node" class="VI" method="Run VI"(reference=w462, error in=w461, "Wait until done"=FALSE ("Wait Until Done"), "Auto Dispose Ref"=FALSE ("Auto Dispose Reference")) -> (error out=w460:errorcluster)  [unwired: 1 in, 4 out]
      }
      frame "Exit" {
        n240 = Unbundle By Name(w484) -> ("notifiers ref.UI Data"=w483:refnum<notifier>, "notifiers ref.Start DAQ"=w482:refnum<notifier>, "notifiers ref.Start Log"=w479:refnum<notifier>)
        n241 = Release Notifier(notifier=w479, error in (no error)=w478) -> (error out=w477:errorcluster)  [unwired: 1 in, 2 out]
        n242 = Release Notifier(notifier=w482, error in (no error)=w477) -> (error out=w481:errorcluster)  [unwired: 1 in, 2 out]
        n243 = Release Notifier(notifier=w483, error in (no error)=w481) -> (error out=w480:errorcluster)  [unwired: 1 in, 2 out]
        n244 = global write "Global 1.vi" "Start DAQ"(FALSE ("Start DAQ")) -> ()
        n245 = global write "Global 1.vi" "Exit"(TRUE ("Exit")) -> ()
        n246 = call "RT Control FGV.vi"("Enum"=enum16{"Read", "Write"}."Write", "RT Ctrl"=cluster{"RT IP":string, "RT Connect":bool} {"RT IP"="localhost", "RT Connect"=FALSE}) -> ()  [unwired: 9 in, 1 out]
      }
    }
    n247 = call <vilib>:"Clear Errors.vi"("error in (no error)"=w138) -> ("error out"=w139:errorcluster)  [unwired: 5 in, 1 out]
  }
  n248 = call "Network Stream.vi"("Queue Ref"=w15) -> ()  [unwired: 11 in]
  n249 = while {
    tunnel: w22 -> [w531]
    stop <- w530 stop-if-true
    n250 = global read "Global 1.vi" "Start DAQ"() -> (w493:bool)
    n251 = Select(t=200, s=w493, f=-1 ("timeout in ms (-1)")) -> (s? t:f=w491:i32)
    n252 = case shown="0, Default" "Select type" {
      tunnel: [w532 w534 w536] -> w490
      tunnel: enum16{"Read", "Write"}."Read" ("Enum") -> [w533 w535 w537]
      frame 0, Default {
        n253 = call "TC FGV.vi"("Enum"=w533) -> ("AI dataout"=w532:waveform(dbl)[])  [unwired: 10 in]
      }
      frame 1 {
        n254 = call "ACC FGV.vi"("Enum"=w535) -> ("AI dataout"=w534:waveform(dbl)[])  [unwired: 10 in]
      }
      frame 2 {
        n255 = call "Strain FGV.vi"("Enum"=w537) -> ("AI dataout"=w536:waveform(dbl)[])  [unwired: 10 in]
      }
    }
    "ACC,TC,SG" <- w490
    n256 = call "DI FGV.vi"("Enum"=enum16{"Read", "Write"}."Read") -> ("DI Data out"=w495:digitalwaveform[])  [unwired: 10 in]
    n257 = Wait on Notification(notifier=w531, timeout in ms (-1)=w491) -> (error out=w530:errorcluster)  [unwired: 2 in, 3 out]
    n258 = call "DI Waveform to Data UI.vi"("DI Data in"=w495) -> ("Array"=w529:bool[])  [unwired: 10 in]
    n259 = call "AI Waveform to Data UI.vi"("AI dataout"=w490) -> ("data"=w487:dbl[])  [unwired: 9 in, 1 out]
    n260 = Index Array(array=w529) -> (element #1=→"HSS 1":bool, element #2=→"HSS 2":bool, element #3=→"HSS 3":bool, element #4=→"HSS 4":bool, element #5=→"HSS 5":bool, element #6=→"HSS 6":bool, element #7=→"HSS 7":bool, element #8=→"HSS 8":bool, element #9=→"HSS 9":bool, element #10=→"HSS 10":bool)  [unwired: 10 in]
    n261 = call "AI FGV.vi"("Enum"=enum16{"Read", "Write"}."Read") -> ("AI dataout"=w488:waveform(dbl)[])  [unwired: 10 in]
    "ACC,TC,SG 2" <- w488
    n262 = call "AI Waveform to Data UI.vi"("AI dataout"=w488) -> ("data"=w486:dbl[])  [unwired: 9 in, 1 out]
    n263 = Index Array(array=w486) -> (element #1=→"AI_1":dbl, element #2=→"AI_ 2":dbl, element #3=→"AI_ 3":dbl, element #4=→"AI_ 4":dbl, element #5=→"AI_ 5":dbl, element #6=→"AI_ 6":dbl, element #7=→"AI_ 7":dbl, element #8=→"AI_ 8":dbl, element #9=→"AI_ 9":dbl, element #10=→"AI_ 10":dbl)  [unwired: 10 in]
    n264 = Array To Cluster(array=w486) -> ()  [unwired: 1 out]
    n265 = Index Array(array=w487) -> (element #1=→"TC1":dbl, element #2=→"TC_2":dbl, element #3=→"TC_3":dbl, element #4=→"TC_4":dbl, element #5=→"TC_5":dbl, element #6=→"TC_6":dbl, element #7=→"TC_7":dbl, element #8=→"TC_8":dbl, element #9=→"TC_9":dbl, element #10=→"TC_10":dbl)  [unwired: 10 in]
  }
  n266 = while {
    tunnel: w29 -> [w543]
    tunnel: [w542] -> w28
    shift-right: [w541] -> w17
    shift-left: errorcluster {"status"=FALSE, "code"=0, "source"=""} ("error out") -> [w540]
    stop <- w538 stop-if-true
    n267 = event shown="[11] \"tdms\": Value Change" {
      selector: w543 -> [_ _ _ _ _ _ _ _ _ _ _ _ _ _ _ _ _]
      dyn-events: [_ _ _ _ _ _ _ _ _ _ _ _ _ _ _ _ _] -> w542
      timeout: _ -> [_ _ _ _ _ _ _ _ _ _ _ _ _ _ _ _ _]
      tunnel: w540 -> [w545 w548 w565 w572 w576 w579 w588 w594 w607 w624 w628 w630 w634 w656 w663 w671 w690]
      tunnel: [w545 w547 w558 w567 w577 w578 w587 w594 w598 w623 w627 w629 w633 w656 w661 w670 w689] -> w539
      tunnel: [FALSE _ _ _ _ _ _ _ _ _ _ _ _ _ _ w672 w691] -> w538
      event Timeout {
        n268 = event-data() -> ()  [unwired: 1 in, 3 out]
      }
      event "Activate Task": Value Change {
        n269 = event-data() -> ("NewVal"=w553:T3)  [unwired: 1 in]
        n270 = Cluster To Array(cluster=w553) -> (array=w552:bool[])
        n271 = Or Array Elements(Boolean array=w552) -> (logical OR=w551:bool)
        n272 = Select(t=T10."Enabled" ("Disabled"), s=w551, f=T10."Disabled and Grayed Out" ("Disabled")) -> (s? t:f=w546:T10)
        n273 = property on="*Select Hardware Configuration File" class="CmbBox"(error in=w548, "DisabledEnum"=w546) -> (error out=w547:errorcluster)  [unwired: 1 in, 1 out]
      }
      event "*Select Hardware Configuration File": Value Change {
        n274 = event-data() -> ("NewVal"=w563:string)  [unwired: 1 in]
        n275 = Empty String/Path?(string/path=w563) -> (empty?=w560:bool)
        n276 = call "Main Queue Driver.vi"("Option"=T9."EnQ '1'", "error in (no error)"=w565, "Message"=cluster{"Message":string, "Data":variant} {"Message"="Load_Config", "Data"=variant}) -> ("error out"=w559:errorcluster)  [unwired: 7 in, 1 out]
        n277 = control-ref of="Start DAQ"() -> (w554:refnum<vi>)
        n278 = Select(t=T10."Disabled and Grayed Out" ("Disabled"), s=w560, f=T10."Enabled" ("Disabled")) -> (s? t:f=w555:T10)
        n279 = call "Boolean Single ref.vi"("controls"=w554, "Enum"=T12."Controls", "Visible"=TRUE, "Disabled"=w555, "error in (no error)"=w559) -> ("error out"=w558:errorcluster)  [unwired: 8 in, 2 out]
      }
      event "Start DAQ": Value Change {
        n280 = event-data() -> ("NewVal"=w568:bool)  [unwired: 1 in]
        n281 = Select(t=cluster{"Message":string, "Data":variant}[] [{"Message"="Load_Config", "Data"=variant}, {"Message"="Rename_Label", "Data"=variant}, {"Message"="Button Logic", "Data"=variant}, {"Message"="Update_AO", "Data"=variant}, {"Message"="Update_DO", "Data"=variant}, {"Message"="Write_DO", "Data"=variant}, {"Message"="Write_AO", "Data"=variant}, {"Message"="Start_DAQ", "Data"=variant}, {"Message"="Selected_type", "Data"=variant}, {"Message"="RTD_graph", "Data"=variant}] ("Message"), s=w568, f=cluster{"Message":string, "Data":variant}[] [{"Message"="Stop_DAQ", "Data"=variant}] ("Message")) -> (s? t:f=w570:cluster{"Message":string, "Data":variant}[])
        n282 = call "Main Queue Driver.vi"("Option"=T9."EnQ 'n'", "error in (no error)"=w572, "Messages"=w570) -> ("error out"=w567:errorcluster)  [unwired: 7 in, 1 out]
      }
      event "Valve_1", "Valve_ 2", "Valve_ 3", "Valve_ 4", "Valve_ 5", "Valve_ 6", "Valve_ 7", "Valve_ 8", "Valve_ 9", "Valve_10": Value Change {
        n283 = event-data() -> ()  [unwired: 1 in, 1 out]
        n284 = call "Main Queue Driver.vi"("Option"=T9."EnQ '1'", "error in (no error)"=w576, "Message"=cluster{"Message":string, "Data":variant} {"Message"="Write_DO", "Data"=variant}) -> ("error out"=w577:errorcluster)  [unwired: 7 in, 1 out]
      }
      event "Update AO": Value Change {
        n285 = event-data() -> ()  [unwired: 1 in, 6 out]
        n286 = call "Main Queue Driver.vi"("Option"=T9."EnQ '1'", "error in (no error)"=w579, "Message"=cluster{"Message":string, "Data":variant} {"Message"="Write_AO", "Data"=variant}) -> ("error out"=w578:errorcluster)  [unwired: 7 in, 1 out]
      }
      event "Start Datalog": Value Change {
        n287 = event-data() -> ("NewVal"=w582:bool)  [unwired: 1 in]
        n288 = global write "Global 1.vi" "Log"(w582) -> ()
        n289 = Select(t=cluster{"Message":string, "notification":bool} {"Message"="Start_Datalog", "notification"=TRUE} ("Message"), s=w582, f=cluster{"Message":string, "notification":bool} {"Message"="Stop_Datalog", "notification"=FALSE} ("Message")) -> (s? t:f=w585:cluster{"Message":string, "notification":bool})
        n290 = call "Main Queue Driver.vi"("Option"=T9."EnQ '1'", "error in (no error)"=w588, "Message"=w585) -> ("error out"=w587:errorcluster)  [unwired: 7 in, 1 out]
      }
      event "Datalog Title:": Value Change {
        # "Update While Typing"
        n291 = event-data() -> ()  [unwired: 1 in, 4 out]
        n292 = global read "Global 1.vi" "Log"() -> (w595:bool)
        n293 = case shown="True" w595 {
          frame False {
          }
          frame True {
            n294 = global write "Global 1.vi" "Restart Log"(TRUE ("Restart Log")) -> ()
          }
        }
        n295 = global write "Global 1.vi" "Datalog"("Datalog Title:") -> ()
        n296 = Empty String/Path?(string/path="Datalog Title:") -> (empty?=w589:bool)
        n297 = Select(t=T10."Disabled and Grayed Out" ("Disabled"), s=w589, f=T10."Enabled" ("Disabled")) -> (s? t:f=w593:T10)
        n298 = property on="Start Datalog" class="Bool (strict)"("DisabledEnum"=w593) -> ()  [unwired: 2 in, 2 out]
      }
      event "Listbox": Value Change {
        n299 = event-data() -> ("NewVal"=w606:i32)  [unwired: 1 in]
        n300 = control-ref of="Tab Control"() -> (w608:refnum<vi>)
        n301 = property on="Property Node" class="TabCtl (strict)"(reference=w608, error in=w607, "Value"=w606) -> (error out=w605:errorcluster, "Value"=w601:T1)  [unwired: 1 out]
        n302 = local read "vi reference"() -> (w604:refnum<vi>)
        n303 = Equal?(x=T1."Hardware Configuration" ("Value"), y=w601) -> (x = y?=w603:bool)
        n304 = case shown="True" w603 {
          tunnel: [w611 w613] -> w597
          tunnel: w605 -> [w612 w613]
          tunnel: w604 -> [w610 _]
          tunnel: [cluster{"Message":string, "Data":variant} {"Message"="Refresh_files", "Data"=variant} ("Message") cluster{"Message":string, "Data":variant} {"Message"="Hardware_config", "Data"=variant} ("Message")] -> w599
          frame False {
            n305 = Close Reference(reference=w610, error in (no error)=w612) -> (error out=w611:errorcluster)
          }
          frame True {
          }
        }
        n306 = call "Main Queue Driver.vi"("Option"=T9."EnQ '1'", "error in (no error)"=w597, "Message"=w599) -> ("error out"=w598:errorcluster)  [unwired: 7 in, 1 out]
      }
      event "Select type": Value Change {
        n307 = event-data() -> ("NewVal"=w619:u16)  [unwired: 1 in]
        n308 = To Variant(anything=w619) -> (Variant=w618:variant)
        n309 = Bundle By Name(cluster=cluster{"Message":string, "Data":variant} {"Message"="Selected_type", "Data"=variant} ("Message"), "Message"="Selected_type", "Data"=w618) -> (w617:cluster{"Message":string, "Data":variant})
        n310 = Build Array(w617, cluster{"Message":string, "Data":variant} {"Message"="Button Logic", "Data"=variant} ("Message")) -> (w615:cluster{"Message":string, "Data":variant}[])
        n311 = call "Main Queue Driver.vi"("Option"=T9."EnQ 'n'", "error in (no error)"=w624, "Messages"=w615) -> ("error out"=w623:errorcluster)  [unwired: 7 in, 1 out]
      }
      event "SEQ": Value Change {
        n312 = event-data() -> ()  [unwired: 1 in, 1 out]
        n313 = call "Main Queue Driver.vi"("Option"=T9."EnQ '1'", "error in (no error)"=w628, "Message"=cluster{"Message":string, "Data":variant} {"Message"="Sequencer", "Data"=variant}) -> ("error out"=w627:errorcluster)  [unwired: 7 in, 1 out]
      }
      event "tdms": Value Change {
        n314 = event-data() -> ()  [unwired: 1 in, 6 out]
        n315 = call <vilib>:"TDMS - File Viewer (NXG Style).vi"("error in"=w630) -> ("error out"=w629:errorcluster)  [unwired: 9 in, 1 out]
      }
      event "RT connect": Value Change {
        n316 = event-data() -> ()  [unwired: 1 in, 5 out]
        n317 = case shown="False" "RT connect" {
          tunnel: w634 -> [w640 w652]
          tunnel: [w640 w645] -> w633
          tunnel: [T10."Enabled" ("f") w641] -> w631
          frame False {
          }
          frame True {
            n318 = call <vilib>:"Set Busy.vi"("error in (no error)"=w652) -> ("error out"=w647:errorcluster)  [unwired: 9 in, 1 out]
            n319 = call "Connection Wait.vi"("error in"=w647, "wait(ms)"=u32 5000) -> ("error  out"=w646:errorcluster, "Status Out"=w642:bool)  [unwired: 8 in]
            n320 = call <vilib>:"Unset Busy.vi"("error in (no error)"=w646) -> ("error out"=w645:errorcluster)  [unwired: 10 in]
            n321 = Select(t=T10."Disabled and Grayed Out" ("Disabled"), s=w642, f=T10."Enabled") -> (s? t:f=w641:T10)
            n322 = Select(t="Successfully connected." ("message"), s=w642, f="Connect to RT failed!" ("T button name (\"OK\")")) -> (s? t:f=w649:string)
            n323 = One Button Dialog(message=w649) -> ()  [unwired: 1 in, 1 out]
          }
        }
        n324 = Bundle(cluster=cluster{"RT IP":string, "RT Connect":bool} {"RT IP"="", "RT Connect"=FALSE} ("RT Ctrl out"), "RT IP"="Target IP Address:", "RT Connect"="RT connect") -> (w637:cluster{"RT IP":string, "RT Connect":bool})
        n325 = call "RT Control FGV.vi"("Enum"=enum16{"Read", "Write"}."Write", "RT Ctrl"=w637) -> ()  [unwired: 9 in, 1 out]
        n326 = property on="File transfer" class="Clust"("DisabledEnum"=w631) -> ()  [unwired: 2 in, 2 out]
      }
      event "Enter Time(period)": Value Change {
        n327 = event-data() -> ()  [unwired: 1 in, 5 out]
        n328 = Multiply(x="Enter Time(period)", y=60.0) -> (x*y=w653:dbl)
        n329 = global write "Global 1.vi" "Log Period"(w653) -> ()
      }
      event "File transfer.sent file": Value Change {
        n330 = event-data() -> ()  [unwired: 1 in, 5 out]
        n331 = call <vilib>:"Set Busy.vi"("error in (no error)"=w663) -> ("error out"=w662:errorcluster)  [unwired: 9 in, 1 out]
        n332 = call "scp_file_transfer.vi"("File transfer 2"="File transfer", "error in (no error)"=w662) -> ("file status"=w660:bool, "File transfer 3"=w658:T2, "error out"=w659:errorcluster)  [unwired: 11 in]
        n333 = property on="File status" class="Bool (strict)"("Value"=w660) -> ()  [unwired: 2 in, 2 out]
        n334 = call "Restart cRIO.vi"("error in (no error)"=w659, "File transfer"=w658) -> ("error out"=w657:errorcluster)  [unwired: 9 in]
        n335 = flat-sequence {
          tunnel: [w667] -> w661
          tunnel: w657 -> [w665]
          frame #0 {
            n336 = call <vilib>:"Unset Busy.vi"() -> ("error out"=w666:errorcluster)  [unwired: 11 in]
            n337 = Merge Errors(w666, w665) -> (w667:errorcluster)
          }
        }
      }
      event "Exit": Value Change {
        n338 = event-data() -> ()  [unwired: 1 in, 1 out]
        n339 = Two Button Dialog ("Confirm Quit")(message="Do you want to Quit Compact Accquistion Software?\n*Note:Confirm DAQ and Datalog Stopped.") -> (T button?=w669:bool)  [unwired: 2 in]
        n340 = case shown="True" w669 {
          tunnel: [FALSE ("Exit") TRUE ("Exit")] -> w672
          tunnel: w671 -> [w674 w686]
          tunnel: [w674 w678] -> w670
          frame False {
          }
          frame True {
            n341 = call "Main Queue Driver.vi"("Option"=T9."EnQ '1'", "error in (no error)"=w686, "Message"=cluster{"Message":string, "Data":variant} {"Message"="Exit", "Data"=variant}) -> ("error out"=w683:errorcluster)  [unwired: 7 in, 1 out]
            n342 = local read "vi reference"() -> (w681:refnum<vi>)
            n343 = To Variant(anything=TRUE ("Exit")) -> (Variant=w676:variant)
            n344 = call "Networkstream UI Command.vi"("error in"=w683, "Data"=w676, "Message"="Exit") -> ("error out"=w679:errorcluster)  [unwired: 8 in]
            n345 = Close Reference(reference=w681) -> (error out=w680:errorcluster)  [unwired: 1 in]
            n346 = Merge Errors(w680, w679) -> (w678:errorcluster)
          }
        }
      }
      event Panel Close? {
        n347 = event-data() -> ()  [unwired: 1 in, 4 out]
        n348 = Two Button Dialog ("Confirm Quit")(message="Do you want to Quit Compact Accquistion Software?\n*Note:Confirm DAQ and Datalog Stopped.") -> (T button?=w688:bool)  [unwired: 2 in]
        n349 = case shown="True" w688 {
          tunnel: [FALSE ("Exit") TRUE ("Exit")] -> w691
          tunnel: w690 -> [w693 w705]
          tunnel: [w693 w697] -> w689
          frame False {
          }
          frame True {
            n350 = call "Main Queue Driver.vi"("Option"=T9."EnQ '1'", "error in (no error)"=w705, "Message"=cluster{"Message":string, "Data":variant} {"Message"="Exit", "Data"=variant}) -> ("error out"=w702:errorcluster)  [unwired: 7 in, 1 out]
            n351 = local read "vi reference"() -> (w700:refnum<vi>)
            n352 = To Variant(anything=TRUE ("Exit")) -> (Variant=w695:variant)
            n353 = call "Networkstream UI Command.vi"("error in"=w702, "Data"=w695, "Message"="Exit") -> ("error out"=w698:errorcluster)  [unwired: 8 in]
            n354 = Close Reference(reference=w700) -> (error out=w699:errorcluster)  [unwired: 1 in]
            n355 = Merge Errors(w699, w698) -> (w697:errorcluster)
          }
        }
        n356 = event-data() -> ()  [unwired: 2 in, 1 out]
      }
    }
    n357 = call <vilib>:"Clear Errors.vi"("error in (no error)"=w539) -> ("error out"=w541:errorcluster)  [unwired: 5 in, 1 out]
  }
  n358 = Destroy User Event(user event=w1, error in=w27) -> (error out=w8:errorcluster)
  n359 = Unregister For Events(event registration refnum=w28, error in=w17) -> (error out=w7:errorcluster)
  n360 = Merge Errors(w7, w8) -> (w6:errorcluster)
  n361 = call <vilib>:"Clear Errors.vi"("error in (no error)"=w6) -> ("error out"=w2:errorcluster)  [unwired: 5 in, 1 out]
  n362 = property class="App"(error in=w2) -> ("App.Kind"=w5:T4)  [unwired: 1 in, 2 out]
  n363 = Equal?(x=w5, y=T4."Run Time System") -> (x = y?=w3:bool)
  n364 = case shown="True" w3 {
    frame False {
    }
    frame True {
      n365 = Quit LabVIEW(quit? (T)=TRUE) -> ()
    }
  }
